vi "Horizontal.vi"(7 "Offset Time":dbl, 8 "error in":errorcluster, 9 "Sample Time":dbl=1.0, 10 "Sample Points":u32=1000, 11 "Instrument Handle In":i32) -> (0 "error out":errorcluster, 3 "Instrument Handle Out":i32)   [LabVIEW 2020, in "ZTScopeM.lvlib"]
doc: "Configure the horizontal and timebase settings."
uses:
  ZTScopeM.lvlib
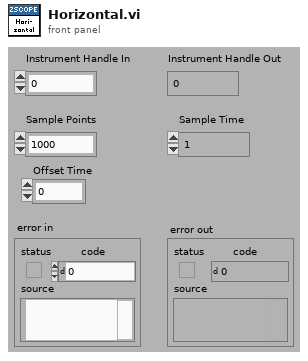
[diagram p1: front panel]
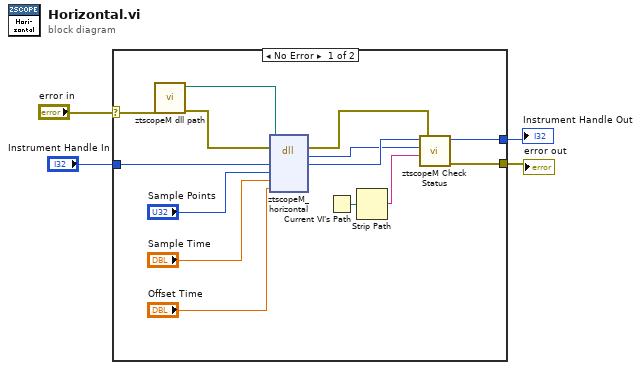
[diagram p0: block diagram]
diagram:
  n1 = case shown="No Error" "error in" {
    selector: "error in" -> [w8 w20]
    tunnel: [w11 w20] -> w1
    tunnel: "Instrument Handle In" -> [w18 w19]
    tunnel: [w10 w19] -> w3
    frame No Error {
      n2 = call "ztscopeM dll path.vi"("error in (no error)"=w8) -> ("error out"=w6:errorcluster, "<instrument>.dll path"=w7:path)  [unwired: 9 in]
      n3 = dll-call lib="C:/Program Files (x86)/National Instruments/LabVIEW 2013/instr.lib/ztscopem/ztscopeM.dll" fn="ztscopeM_horizontal"(path in=w7, error in=w6, "instrumentHandle"=w18, "samplePoints"="Sample Points", "sampleTime"="Sample Time", "offsetTime"="Offset Time") -> (error out=w5:errorcluster, w12:i32, "instrumentHandle"=w13:i32)  [unwired: 4 in, 1 out]
      n4 = Current VI's Path() -> (path=w15:path)
      n5 = Strip Path(path=w15) -> (name=w14:string)  [unwired: 1 out]
      n6 = call "ztscopeM Check Status.vi"("error in"=w5, "name of VI"=w14, "status (return code)"=w12, "instrument handle in"=w13) -> ("error out"=w11:errorcluster, "instrument handle out"=w10:i32)  [unwired: 2 in]
    }
    frame Error {
    }
  }
  "Instrument Handle Out" <- w3
  "error out" <- w1
